vi "Pause.vi"(8 "error in (no error)":errorcluster, 11 "VICI Settings":T1 {"Pump Number" min=0.0 max=20.0 step=1.0}) -> (0 "error out":errorcluster, 3 "VICI Settings":T1 {"Pump Number" min=0.0 max=20.0 step=1.0})   [LabVIEW 2018, in "VICI M50.lvlib"]
uses:
  VICI M50.lvlib
  Settings Cluster.ctl
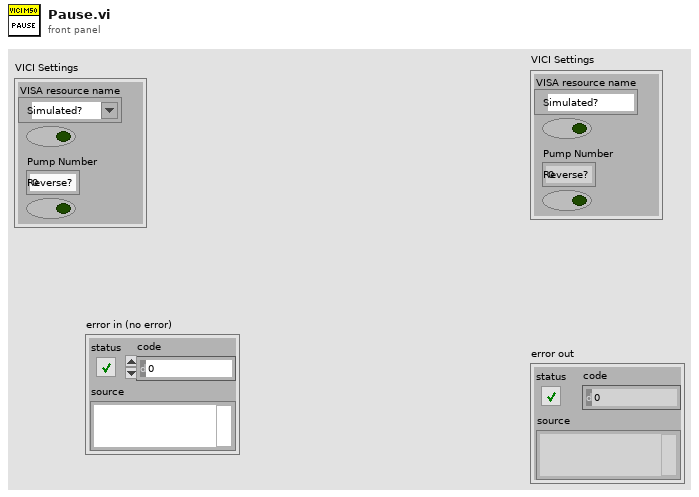
[diagram p1: front panel]
types:
  T1 = typedef "VICI M50.lvlib/Settings Cluster.ctl" = cluster{"VISA resource name":refnum<visa-resource-name>, "Simulated?":bool, "Pump Number":dbl, "Reverse?":bool}
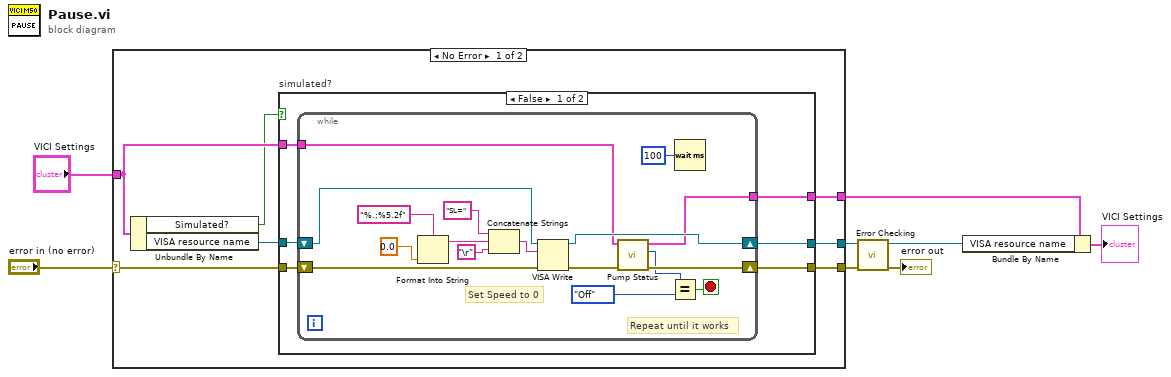
[diagram p0: block diagram]
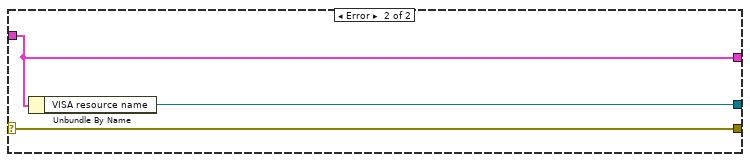
[diagram p3: hidden frame]
diagram:
  n1 = case shown="No Error" "error in (no error)" {
    selector: "error in (no error)" -> [w15 w44]
    tunnel: [w11 w43] -> w2
    tunnel: "VICI Settings" -> [w12 w43]
    tunnel: [w14 w42] -> w6
    tunnel: [w13 w44] -> w5
    frame No Error {
      n2 = Unbundle By Name(w12) -> ("Simulated?"=w9:bool, "VISA resource name"=w10:refnum<visa-resource-name>)
      n3 = case "simulated?" shown="False" w9 {
        tunnel: [w19 w41] -> w14
        tunnel: w10 -> [w21 w41]
        tunnel: w15 -> [w20 w40]
        tunnel: [w18 w40] -> w13
        tunnel: w12 -> [w17 w39]
        tunnel: [w16 w39] -> w11
        frame False {
          n4 = while {
            shift-right: [w36] -> w19
            shift-left: w21 -> [w38]
            shift-right: [w28] -> w18
            shift-left: w20 -> [w37]
            tunnel: w17 -> [w27]
            tunnel: [w26] -> w16
            stop <- w22 stop-if-true
            # "Repeat until it works"
            # "Set Speed to 0"
            n5 = Format Into String(format string="%.;%5.2f", 0.0 ("input 1")) -> (resulting string=w34:string)  [unwired: 2 in, 1 out]
            n6 = Concatenate Strings("SL=" ("string"), w34, "\r") -> (w33:string)
            n7 = VISA Write(VISA resource name=w38, write buffer=w33, error in (no error)=w37) -> (VISA resource name out=w36:refnum<visa-resource-name>, error out=w29:errorcluster)  [unwired: 1 out]
            n8 = call "Pump Status.vi"("error in (no error)"=w29, "VICI Settings"=w27) -> ("error out"=w28:errorcluster, "Pump On?"=w24:enum16{"Off", "On", "Not Initialized"}, "VICI Settings"=w26:T1)  [unwired: 6 in, 1 out]
            n9 = Equal?(x=w24, y=enum16{"Off", "On", "Not Initialized"}."Off") -> (x = y?=w22:bool)
            n10 = Wait (ms)(milliseconds to wait=u32 100) -> ()  [unwired: 1 out]
          }
        }
        frame True {
        }
      }
    }
    frame Error {
      n11 = Unbundle By Name(w43) -> ("VISA resource name"=w42:refnum<visa-resource-name>)
    }
  }
  n12 = call "Error Checking.vi"("error in (no error)"=w5, "VISA resource name"=w6) -> ("error out"=→"error out":errorcluster, "VISA resource name"=w3:refnum<visa-resource-name>)  [unwired: 7 in, 1 out]
  n13 = Bundle By Name(cluster=w2, "VISA resource name"=w3) -> (→"VICI Settings":T1)
